vi "ActionVIOnDownload.vi"(5 "System Definition Dir":path, 6 "IP address":string, 7 "Details Ref":refnum<vi>, 8 "error in (no error)":errorcluster, 10 "WebDAV session in":T1, 11 "Device Item Ref in":T2 format="%.0x") -> (0 "error out":errorcluster, 2 "WebDAV session out":T1, 3 "Device Item Ref out":T2 format="%.0x")   [LabVIEW 2020, in "Communication Bus Template System Explorer.lvlib" / "Implementation.lvlib"]
uses:
  Implementation.lvlib
  Scripting/Communication Bus Template Scripting.lvlib
  C:/Program Files (x86)/National Instruments/VeriStand 2020/NationalInstruments.VeriStand.ServerAPI.dll
  Program Files (x86)/National Instruments/VeriStand 2020/NationalInstruments.VeriStand.ServerAPI.dll
  <vilib>/NI VeriStand/Custom Device Tools/Custom Device Utility Library/Custom Device Utility Library.lvlib
  Scripting/Constants.vi
  <vilib>/NI VeriStand/Custom Device Tools/Custom Device Utility Library/NI VeriStand - Search for Item by GUID.vi
  <vilib>/NI VeriStand/Custom Device API/Custom Device Item Ref.ctl
  <vilib>/NI VeriStand/Custom Device API/Custom Device API.lvlib
  <vilib>/WebDAVClient/Advanced/SessionHandle.ctl
  <vilib>/WebDAVClient/NI_WebDAV.lvlib
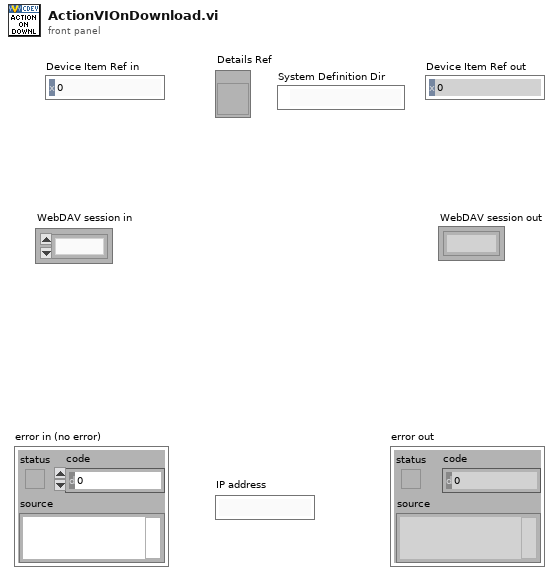
[diagram p1: front panel]
types:
  T1 = typedef "NI_WebDAV.lvlib/SessionHandle.ctl" = refnum<k1>
  T2 = typedef "Custom Device API.lvlib/Custom Device Item Ref.ctl" = u64
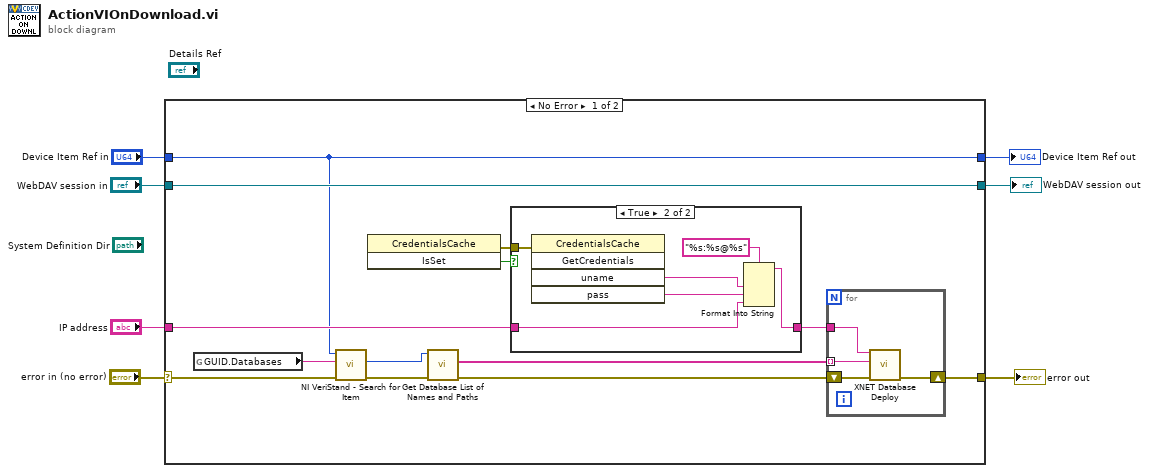
[diagram p0: block diagram]
diagram:
  n1 = case shown="No Error" "error in (no error)" {
    selector: "error in (no error)" -> [w12 w34]
    tunnel: [w19 w34] -> w6
    tunnel: "WebDAV session in" -> [w20 w33]
    tunnel: [w20 w33] -> w2
    tunnel: "Device Item Ref in" -> [w8 w32]
    tunnel: [w8 w32] -> w4
    tunnel: "IP address" -> [w14 _]
    frame No Error {
      n2 = global read "Constants.vi" "GUID.Databases"() -> (w9:string)
      n3 = call-poly <vilib>:"NI VeriStand - Search for Item.vi"("error in"=w12, "Item GUID"=w9, "Section Ref in"=w8) -> ("error out"=w11:errorcluster, "Item Ref"=w10:T2)  [unwired: 5 in, 2 out]
      n4 = invoke class="CredentialsCache" method="IsSet"() -> (error out=w16:errorcluster, "IsSet"=w15:bool)  [unwired: 3 in, 1 out]
      n5 = call "Get Database List of Names and Paths.vi"("error in"=w11, "Databases section Ref"=w10) -> ("error out"=w18:errorcluster, "Names"=w17:string[])  [unwired: 6 in, 2 out]
      n6 = case shown="True" w15 {
        tunnel: w16 -> [_ w27]
        tunnel: w14 -> [w21 w23]
        tunnel: [w21 w22] -> w13
        frame False {
        }
        frame True {
          n7 = invoke class="CredentialsCache" method="GetCredentials"(error in=w27) -> ("uname"=w25:string, "pass"=w24:string)  [unwired: 4 in, 3 out]
          n8 = Format Into String(format string="%s:%s@%s", w25, w24, w23) -> (resulting string=w22:string)  [unwired: 2 in, 1 out]
        }
      }
      n9 = for {
        shift-right: [w31] -> w19
        shift-left: w18 -> [w30]
        tunnel: w17 -> [w29] mode=indexing
        tunnel: w13 -> [w28]
        n10 = call <vilib>:"XNET Database Deploy.vi"("IP address"=w28, "alias"=w29, "error in (no error)"=w30) -> ("error out"=w31:errorcluster)  [unwired: 11 in, 1 out]
      }
    }
    frame Error {
    }
  }
  "error out" <- w6
  "Device Item Ref out" <- w4
  "WebDAV session out" <- w2
